vi "WFLC.vi"(0 "Prediction Lookahead":sgl, 1 "Signal":sgl[](array[numeric]), 2 "u0":dbl=1.67e-05, 5 "i":sgl[](array[numeric]), 7 "sumw0":dbl[](array[numeric]), 9 "w0":dbl[](array[numeric]), 11 "w1":dbl[](array[numeric]), 12 "w2":dbl[](array[numeric]), 13 "u":dbl=0.0167) -> (4 "out i":sgl[](array[numeric]), 6 "out sumw0":dbl[](array[numeric]), 8 "out w0":dbl[](array[numeric]), 10 "out w1":dbl[](array[numeric]), 14 "Prediction":dbl[](array[numeric]), 15 "out w2":dbl[](array[numeric]))   [LabVIEW 2010]
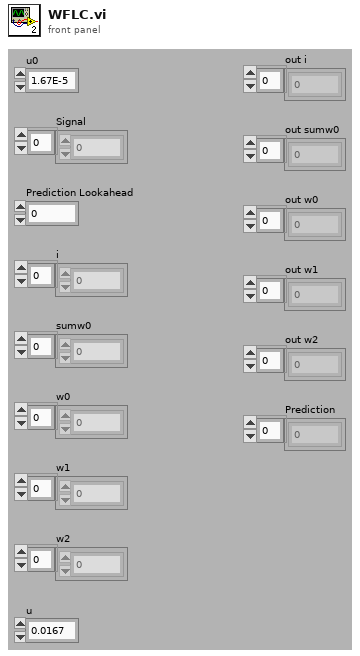
[diagram p1: front panel]
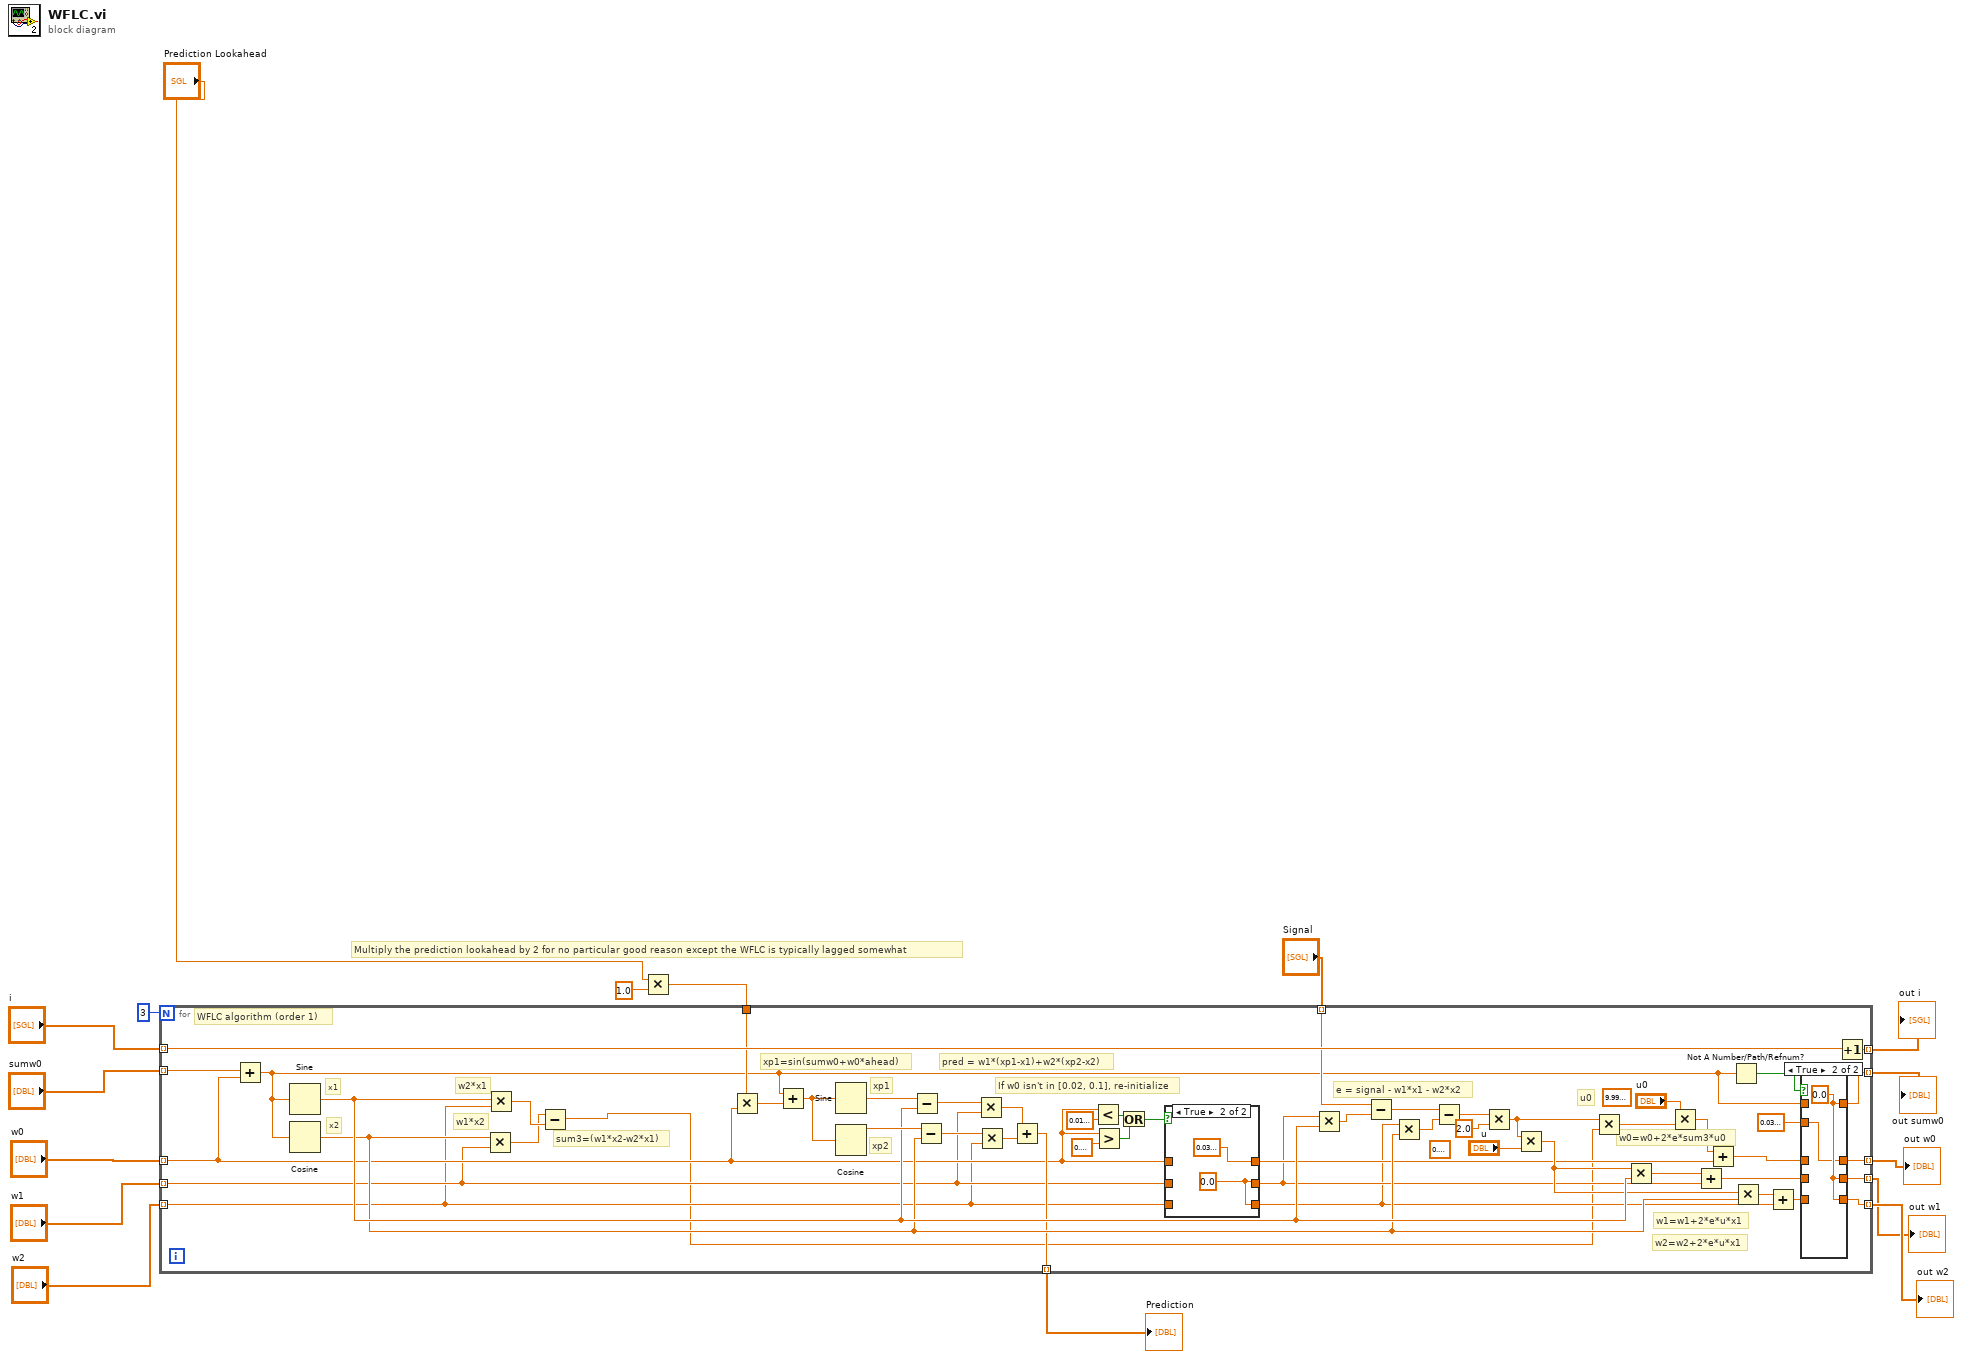
[diagram p0: block diagram]
diagram:
  # "Multiply the prediction lookahead by 2 for no particular good reason except the WFLC is typically lagged somewhat"
  n1 = Multiply(x="Prediction Lookahead", y=sgl 1.0 ("t")) -> (x*y=w1:sgl)
  n2 = for {
    N: 3 ("t") -> [_]
    tunnel: [w69] -> w4 mode=indexing
    tunnel: "sumw0" -> [w68] mode=indexing
    tunnel: "i" -> [w65] mode=indexing
    tunnel: w1 -> [w64]
    tunnel: "Signal" -> [w55] mode=indexing
    tunnel: "w0" -> [w24] mode=indexing
    tunnel: [w38] -> w9 mode=indexing
    tunnel: [w36] -> w10 mode=indexing
    tunnel: "w2" -> [w22] mode=indexing
    tunnel: "w1" -> [w23] mode=indexing
    tunnel: [w34] -> w13 mode=indexing
    tunnel: [w33] -> w14 mode=indexing
    tunnel: [w41] -> w16 mode=indexing
    (unwired) sgl 0.2 ("t")
    (unwired) sgl 0.0001 ("t")
    # "If w0 isn't in [0.02, 0.1], re-initialize"
    # "WFLC algorithm (order 1)"
    # "w2=w2+2*e*u*x1"
    # "w1=w1+2*e*u*x1"
    # "w0=w0+2*e*sum3*u0"
    # "u0"
    # "e = signal - w1*x1 - w2*x2"
    # "pred = w1*(xp1-x1)+w2*(xp2-x2)"
    # "xp2"
    # "xp1"
    # "xp1=sin(sumw0+w0*ahead)"
    # "sum3=(w1*x2-w2*x1)"
    # "w1*x2"
    # "w2*x1"
    # "x2"
    # "x1"
    n3 = Add(x=w68, y=w24) -> (x+y=w39:dbl)
    n4 = Sine(x=w39) -> (sin(x)=w46:dbl)
    n5 = Cosine(x=w39) -> (cos(x)=w43:dbl)
    n6 = Multiply(x=w43, y=w23) -> (x*y=w66:dbl)
    n7 = Multiply(x=w46, y=w22) -> (x*y=w67:dbl)
    n8 = Subtract(x=w66, y=w67) -> (x-y=w17:dbl)
    n9 = Multiply(x=w64, y=w24) -> (x*y=w63:dbl)
    n10 = Add(x=w39, y=w63) -> (x+y=w62:dbl)
    n11 = Sine(x=w62) -> (sin(x)=w61:dbl)
    n12 = Cosine(x=w62) -> (cos(x)=w60:dbl)
    n13 = Subtract(x=w61, y=w46) -> (x-y=w59:dbl)
    n14 = Subtract(x=w60, y=w43) -> (x-y=w58:dbl)
    n15 = Multiply(x=w59, y=w23) -> (x*y=w57:dbl)
    n16 = Multiply(x=w58, y=w22) -> (x*y=w56:dbl)
    n17 = Add(x=w57, y=w56) -> (x+y=w41:dbl)
    n18 = Less?(x=w24, y=sgl 0.02 ("t")) -> (x < y?=w25:bool)
    n19 = Greater?(x=w24, y=sgl 0.1 ("t")) -> (0:w26:bool)
    n20 = Or(x=w25, y=w26) -> (x .or. y?=w18:bool)
    n21 = case shown="True" w18 {
      tunnel: w24 -> [w72 _]
      tunnel: w23 -> [w71 _]
      tunnel: w22 -> [w70 _]
      tunnel: [w72 sgl 0.04 ("t")] -> w21
      tunnel: [w71 w73] -> w20
      tunnel: [w70 w73] -> w19
      frame False {
      }
      frame True {
        w73 = sgl 0.0 ("t")
      }
    }
    n22 = Multiply(x=w20, y=w46) -> (x*y=w53:dbl)
    n23 = Subtract(x=w55, y=w53) -> (x-y=w54:dbl)
    n24 = Multiply(x=w19, y=w43) -> (x*y=w52:dbl)
    n25 = Subtract(x=w54, y=w52) -> (x-y=w51:dbl)
    n26 = Multiply(x=w51, y=sgl 2.0 ("t")) -> (x*y=w47:dbl)
    n27 = Multiply(x=w47, y="u") -> (x*y=w44:dbl)
    n28 = Multiply(x=w47, y=w17) -> (x*y=w49:dbl)
    n29 = Multiply(x=w44, y=w46) -> (x*y=w45:dbl)
    n30 = Multiply(x="u0", y=w49) -> (x*y=w48:dbl)
    n31 = Add(x=w45, y=w20) -> (x+y=w35:dbl)
    n32 = Add(x=w48, y=w21) -> (x+y=w37:dbl)
    n33 = Not A Number/Path/Refnum?(number/path/refnum=w39) -> (NaN/Path/Refnum?=w40:bool)
    n34 = Multiply(x=w44, y=w43) -> (x*y=w42:dbl)
    n35 = Add(x=w42, y=w19) -> (x+y=w32:dbl)
    n36 = case shown="True" w40 {
      tunnel: w39 -> [w78 _]
      tunnel: [w78 w80] -> w38
      tunnel: w37 -> [w77 _]
      tunnel: [w77 w79] -> w36
      tunnel: w35 -> [w76 _]
      tunnel: [w76 w80] -> w34
      tunnel: [w75 w80] -> w33
      tunnel: w32 -> [w75 _]
      tunnel: sgl 0.04 ("t") -> [_ w79]
      frame False {
      }
      frame True {
        w80 = sgl 0.0 ("t")
      }
    }
    n37 = Increment(x=w65) -> (x+1=w69:sgl)
  }
  "Prediction" <- w16
  "out w2" <- w14
  "out w1" <- w13
  "out w0" <- w10
  "out sumw0" <- w9
  "out i" <- w4
